vi "SubVI_blueprint.vi"() -> ()   [LabVIEW 2016]
panel:
  in  "stop":bool
  in  "STOP ALL":bool
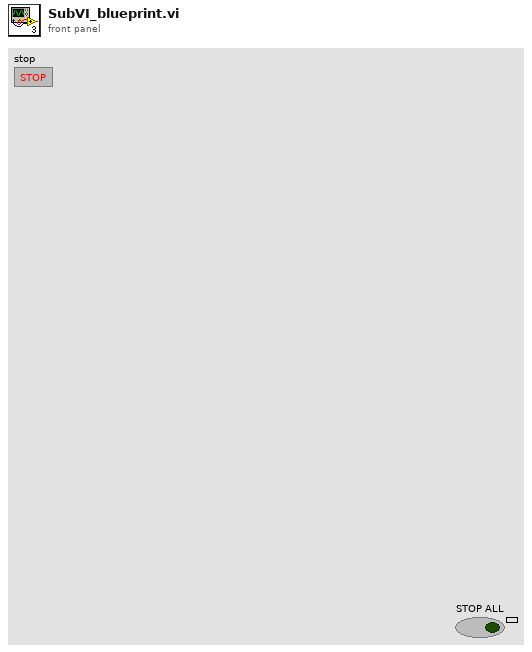
[diagram p1: front panel]
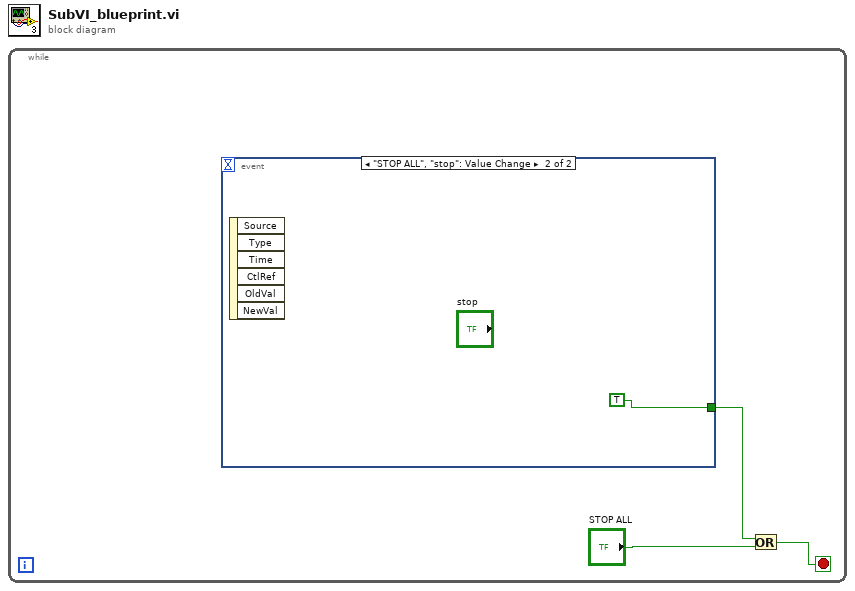
[diagram p0: block diagram]
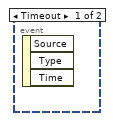
[diagram p2: hidden frame]
diagram:
  n1 = while {
    stop <- w1 stop-if-true
    n2 = event shown="[1] \"STOP ALL\", \"stop\": Value Change" {
      selector: _ -> [_ _]
      dyn-events: _ -> [_ _]
      timeout: _ -> [_ _]
      tunnel: [_ TRUE] -> w2
      event Timeout {
        n3 = event-data() -> ()  [unwired: 1 in, 3 out]
      }
      event "STOP ALL", "stop": Value Change {
        n4 = event-data() -> ()  [unwired: 1 in, 6 out]
      }
    }
    n5 = Or(x=w2, y="STOP ALL") -> (x .or. y?=w1:bool)
  }
